vi "Launcher PC.vi"   [LabVIEW 2021]
panel:
  # "LAUNCHER"
types:
  T1 = enum32{"Invalid", "Standard", "Closed", "Hidden", "Minimized", "Maximized"}
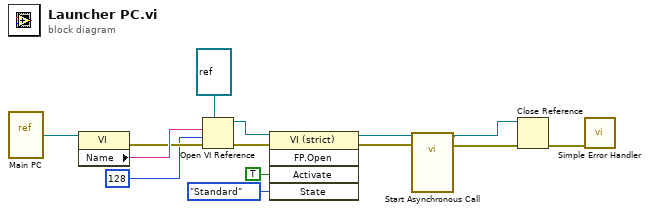
[diagram p0: block diagram]
diagram:
  n1 = vi-ref "Main PC.vi"() -> (w14:refnum<vi>)
  n2 = property class="VI"(reference=w14) -> (error out=w12:errorcluster, "Name"=w13:string)  [unwired: 1 in, 1 out]
  n3 = Open VI Reference(type specifier VI Refnum (for type only)=refnum<vi> refnum, vi path=w13, options=128, error in (no error)=w12) -> (vi reference=w9:refnum<vi>, error out=w10:errorcluster)  [unwired: 2 in]
  n4 = invoke class="VI (strict)" method="FP.Open"(reference=w9, error in=w10, "Activate"=TRUE ("Activate?"), "State"=T1."Standard") -> (reference out=w8:refnum<vi>, error out=w7:errorcluster)  [unwired: 1 in, 3 out]
  n5 = call-by-ref "Start Asynchronous Call"(reference=w8, error in=w7) -> (reference out=w5:refnum<vi>, error out=w6:errorcluster)  [unwired: 12 in]
  n6 = Close Reference(reference=w5, error in (no error)=w6) -> (error out=w4:errorcluster)
  n7 = call <vilib>:"Simple Error Handler.vi"("error in (no error)"=w4) -> ()  [unwired: 4 in, 5 out]
